vi "temporary multiple image tcp example.vi"() -> ()   [LabVIEW 2011]
uses:
  <vilib>/vision/Image Controls.llb/IMAQ Image.ctl
panel:
  out "Image 4":T1(plugin-control)
  out "Image 3":T1(plugin-control)
  out "Image 2":T1(plugin-control)
  in  "stop":bool
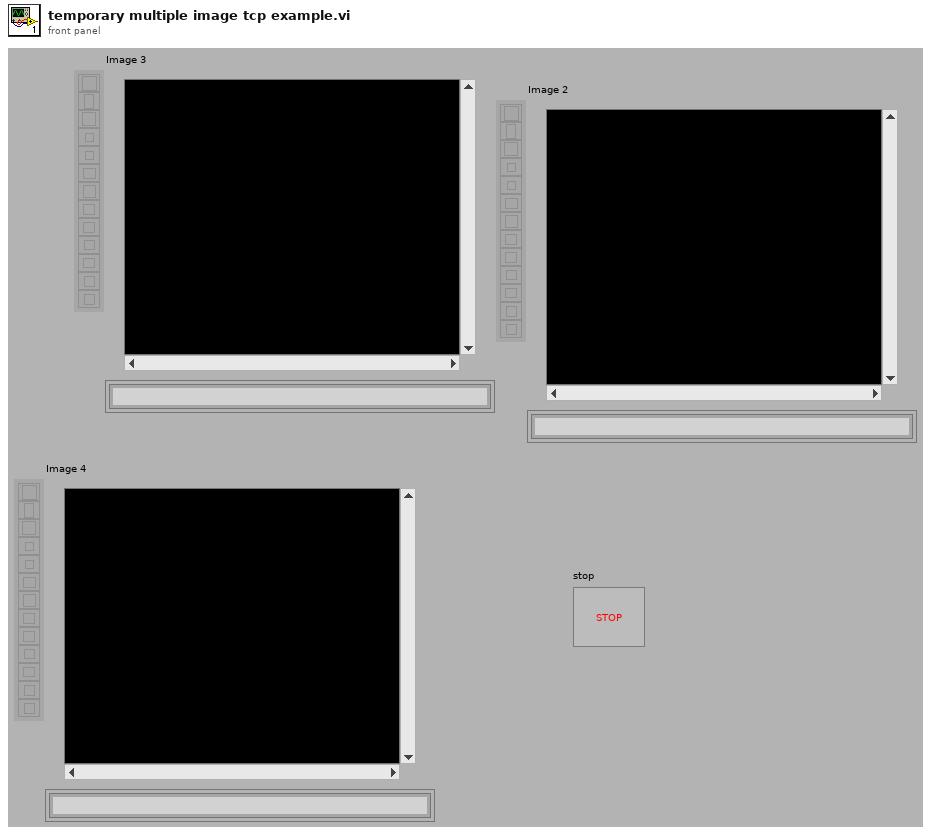
[diagram p1: front panel]
types:
  T1 = typedef "IMAQ Image.ctl" = refnum<image>
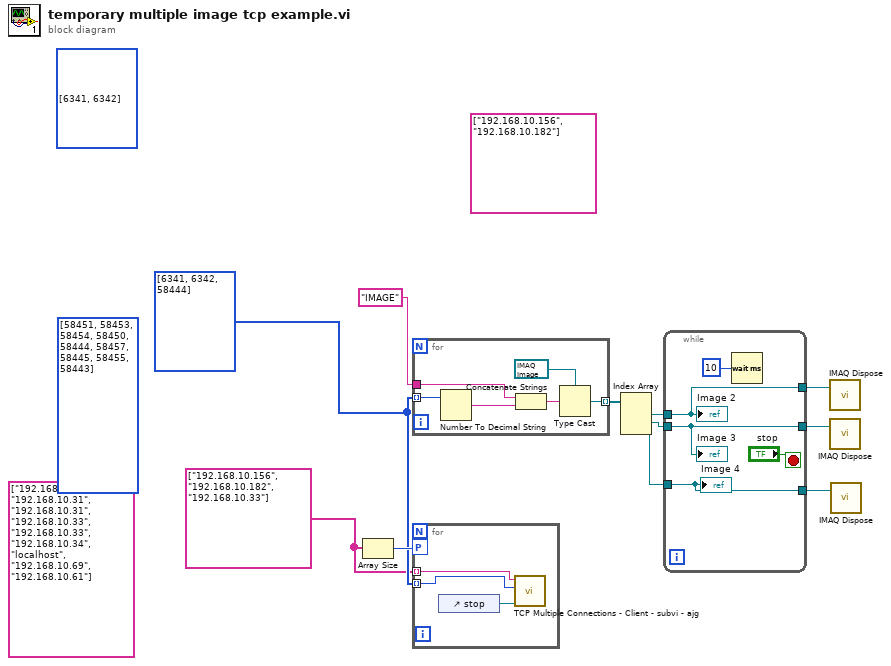
[diagram p0: block diagram]
diagram:
  (unwired) string[] ["192.168.10.156", "192.168.10.182"]
  (unwired) u16[] [6341, 6342]
  (unwired) u16[] [58451, 58453, 58454, 58450, 58444, 58457, 58445, 58455, 58443]
  (unwired) string[] ["192.168.10.151", "192.168.10.31", "192.168.10.31", "192.168.10.33", "192.168.10.33", "192.168.10.34", "localhost", "192.168.10.69", "192.168.10.61"]
  w4 = u16[] [6341, 6342, 58444]
  w3 = string[] ["192.168.10.156", "192.168.10.182", "192.168.10.33"]
  n1 = Array Size(array=w3) -> (size(s)=w11:i32)
  n2 = for {
    tunnel: "IMAGE" ("Image Name") -> [w14]
    tunnel: w4 -> [w13] mode=indexing
    tunnel: [w12] -> w6 mode=indexing
    n3 = Number To Decimal String(number=w13) -> (decimal integer string=w15:string)  [unwired: 1 in]
    n4 = Concatenate Strings(w14, w15) -> (w16:string)
    n5 = Type Cast(type=T1 refnum ("New Image"), x=w16) -> (*(type *) &x=w12:T1)
  }
  n6 = for {
    tunnel: w4 -> [w19] mode=indexing
    tunnel: w3 -> [w20] mode=indexing
    workers-P: w11 -> [_]
    n7 = control-ref of="stop"() -> (w18:refnum<vi>)
    n8 = call "TCP Multiple Connections - Client - subvi - ajg.vi"("stop 2"=w18, "Port"=w19, "Machine"=w20) -> ()  [unwired: 7 in, 2 out]
  }
  n9 = Index Array(array=w6) -> (element #1=w10:T1, element #2=w8:T1, element #3=w2:T1)  [unwired: 3 in]
  n10 = while {
    tunnel: w10 -> [w23]
    tunnel: [w23] -> w9
    tunnel: w8 -> [w22]
    tunnel: [w22] -> w7
    tunnel: w2 -> [w21]
    tunnel: [w21] -> w1
    stop <- "stop" stop-if-true
    n11 = Wait (ms)(milliseconds to wait=u32 10) -> ()  [unwired: 1 out]
    "Image 2" <- w23
    "Image 3" <- w22
    "Image 4" <- w21
  }
  n12 = call "IMAQ Dispose"("Image"=w9) -> ()  [unwired: 5 in, 1 out]
  n13 = call "IMAQ Dispose"("Image"=w7) -> ()  [unwired: 5 in, 1 out]
  n14 = call "IMAQ Dispose"("Image"=w1) -> ()  [unwired: 5 in, 1 out]
